vi "addComplexOne.vi"(8 "error in (no error)":errorcluster, 11 "complexNum":T1) -> (0 "error out":errorcluster, 1 "function return":i32, 3 "complexNumOut":T1)   [LabVIEW 2018]
doc: "Add the complex with one function. This is for the test purpose."
uses:
  typeDef/complexNum.ctl
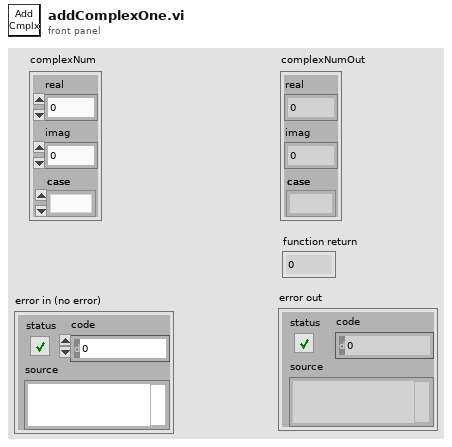
[diagram p1: front panel]
types:
  T1 = typedef "complexNum.ctl" = cluster{"real":dbl, "imag":dbl, "case":enum16{"", "AddOne", "AddTwo"}}
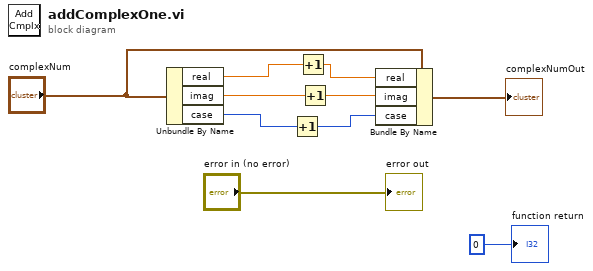
[diagram p0: block diagram]
diagram:
  n1 = Unbundle By Name("complexNum") -> ("real"=w5:dbl, "imag"=w4:dbl, "case"=w2:enum16{"", "AddOne", "AddTwo"})
  n2 = Increment(x=w2) -> (x+1=w1:enum16{"", "AddOne", "AddTwo"})
  n3 = Increment(x=w5) -> (x+1=w9:dbl)
  n4 = Increment(x=w4) -> (x+1=w8:dbl)
  n5 = Bundle By Name(cluster="complexNum", "real"=w9, "imag"=w8, "case"=w1) -> (→"complexNumOut":T1)
  "error out" <- "error in (no error)"
  "function return" <- 0 ("function return")
